vi "Format Into Table Row.vi"(8 "error in (no error)":errorcluster, 11 "Transaction in":refnum<class "Transaction.lvclass">) -> (0 "error out":errorcluster, 3 "Table Row":string[](array[string]))   [LabVIEW 2018, in "Transaction.lvclass"]
uses:
  Transaction.lvclass
  Transaction.lvclass/Transaction.ctl
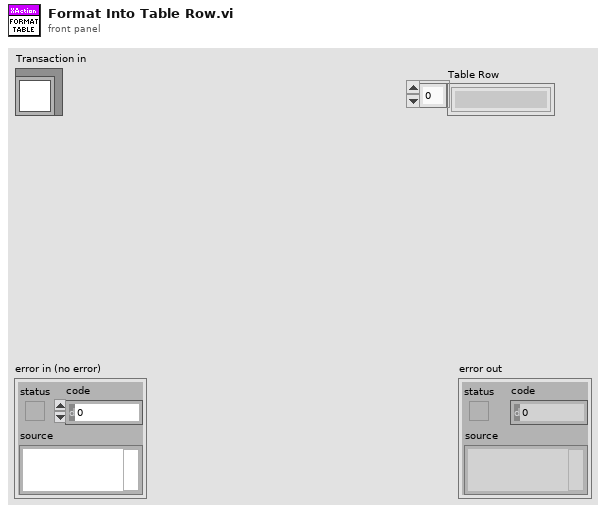
[diagram p1: front panel]
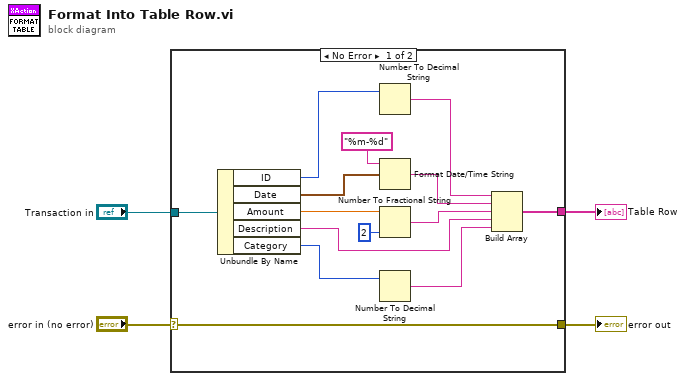
[diagram p0: block diagram]
diagram:
  n1 = case shown="No Error" "error in (no error)" {
    selector: "error in (no error)" -> [w18 w19]
    tunnel: [w18 w19] -> w3
    tunnel: "Transaction in" -> [w17 _]
    tunnel: [w12 _] -> w1
    frame No Error {
      n2 = Unbundle By Name(w17) -> ("ID"=w8:i32, "Date"=w16:timestamp, "Amount"=w11:dbl, "Description"=w9:string, "Category"=w6:i32)
      n3 = Number To Decimal String(number=w8) -> (decimal integer string=w7:string)  [unwired: 1 in]
      n4 = Format Date/Time String(time format string (%c)="%m-%d", seconds (now)=w16) -> (date/time string=w13:string)  [unwired: 1 in]
      n5 = Number To Fractional String(number=w11, precision (6)=i16 2) -> (F-format string=w10:string)  [unwired: 2 in]
      n6 = Number To Decimal String(number=w6) -> (decimal integer string=w5:string)  [unwired: 1 in]
      n7 = Build Array(w7, w13, w10, w9, w5) -> (w12:string[])
    }
    frame Error {
    }
  }
  "error out" <- w3
  "Table Row" <- w1
